vi "SpreadsheetToArrayAndWaveform.vi"(4 "dimension size":i32=600000, 5 "file path (dialog if empty)":path) -> (1 "Waveform Graph":waveform(dbl)(graph), 2 "output array":dbl[](array[numeric]))   [LabVIEW 2015]
uses:
  <vilib>/Utility/file.llb/Read Delimited Spreadsheet (DBL).vi
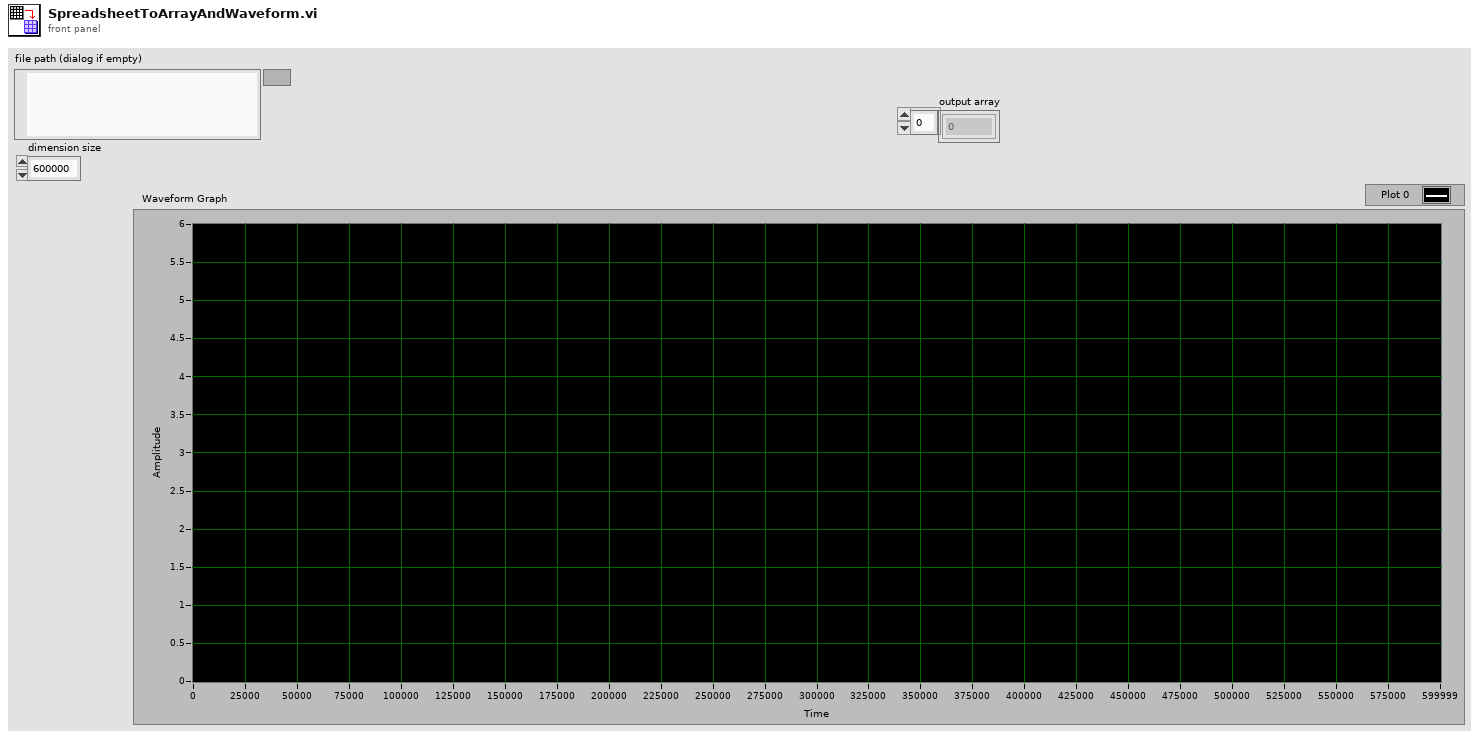
[diagram p1: front panel]
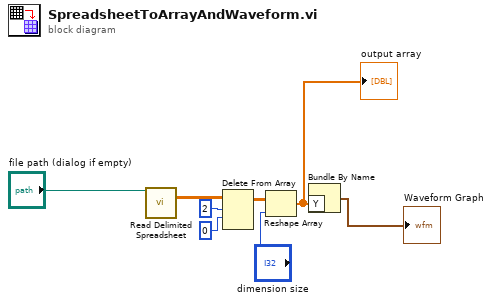
[diagram p0: block diagram]
diagram:
  n1 = call-poly <vilib>:"Read Delimited Spreadsheet.vi"("file path (dialog if empty)"="file path (dialog if empty)") -> ("all rows"=w8:dbl[][])  [unwired: 9 in, 5 out]
  n2 = Delete From Array(array=w8, length=2, index (row)=0) -> (array with subset deleted=w5:dbl[][])  [unwired: 1 in, 1 out]
  n3 = Reshape Array(w5, "dimension size") -> (w3:dbl[])
  "output array" <- w3
  n4 = Bundle By Name("Y"=w3) -> (→"Waveform Graph":waveform(dbl))  [unwired: 1 in]
